vi "MeasureFastJoule.vi"(0 ".NET Refnum in":refnum<k24>, 1 ".NET Refnum":refnum<k24>, 2 "Junction Name":string, 5 "Maxiumum Voltage":dbl=8.0, 7 "appended path":path, 12 "new file path (Not A Path if cancelled)":path, 13 "UiDefinition":T1, 14 "Function":string) -> (15 "error out":errorcluster)   [LabVIEW 2020]
uses:
  D:/LabviewDXFViewer/LabviewDXFViewer/bin/Release/LabviewDXFViewer.exe
  LabviewDXFViewer/bin/Release/LabviewDXFViewer.exe
  UIReferences.ctl
  <vilib>/Utility/file.llb/Write Delimited Spreadsheet (string).vi
  <vilib>/Utility/file.llb/Write Delimited Spreadsheet (DBL).vi
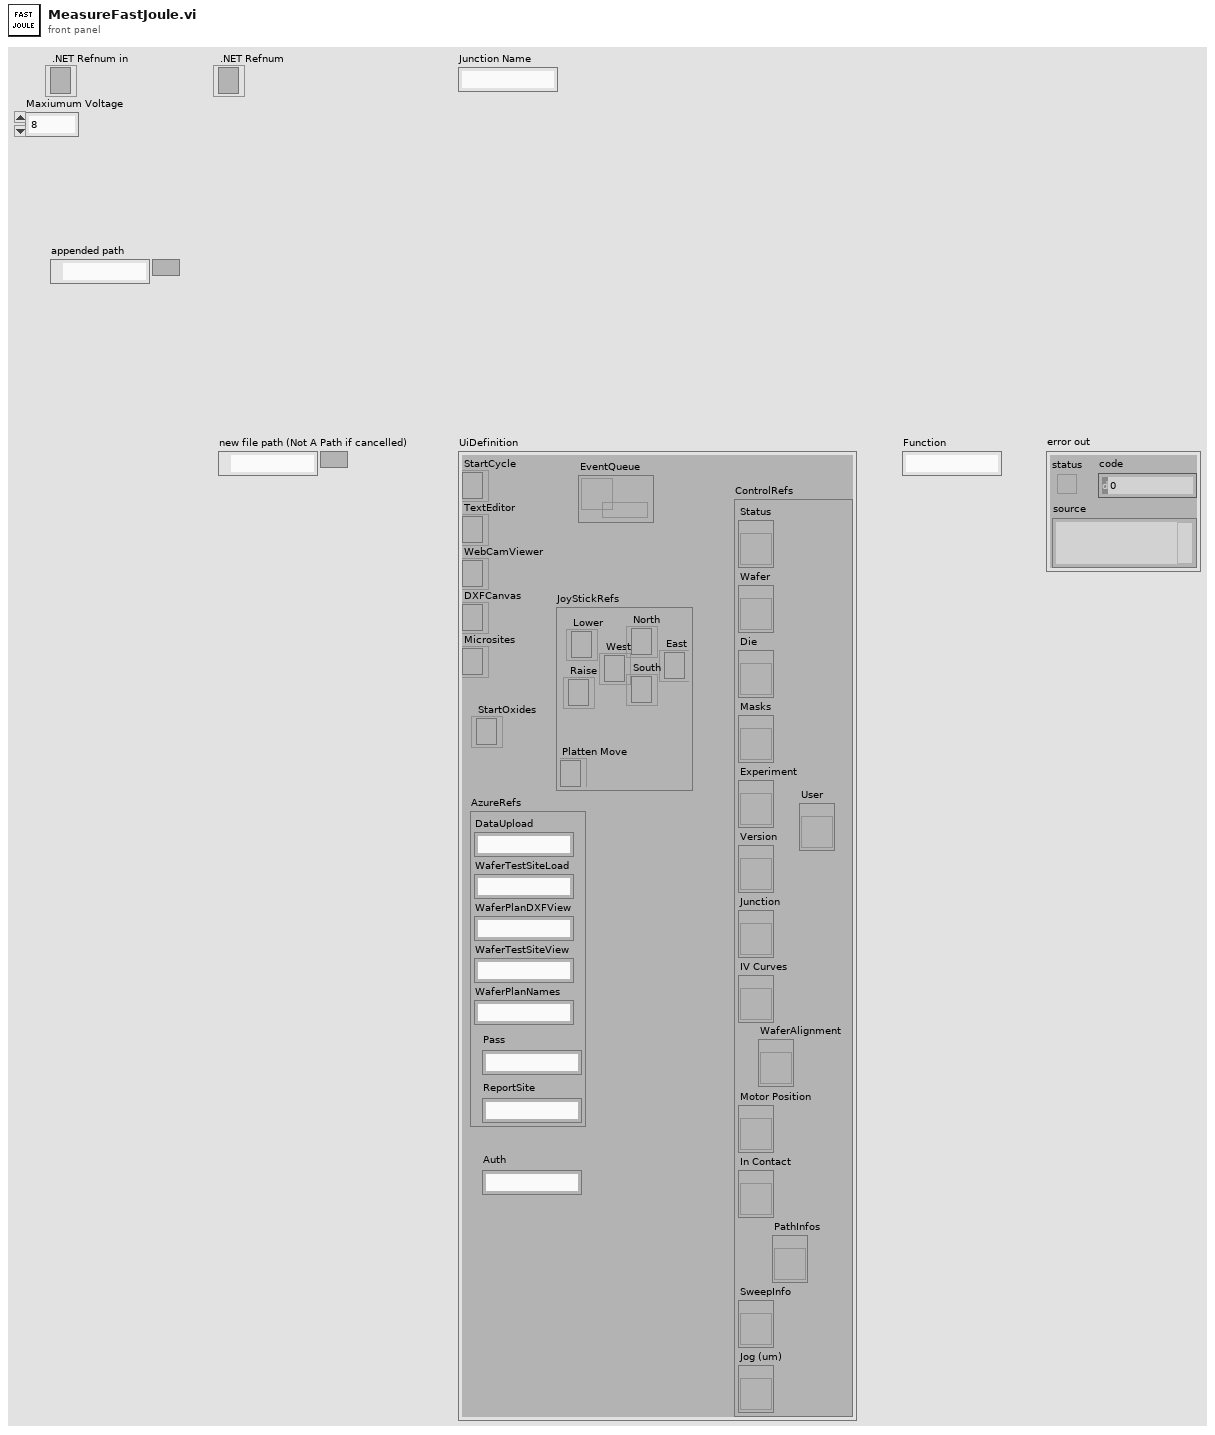
[diagram p1: front panel]
types:
  T1 = typedef "UIReferences.ctl" = cluster{"StartCycle":refnum<k24>, "TextEditor":refnum<k24>, "WebCamViewer":refnum<k24>, "DXFCanvas":refnum<k24>, "Microsites":refnum<k24>, "JoyStickRefs":cluster{"North":refnum<k24>, "Lower":refnum<k24>, "Raise":refnum<k24>, "Platten Move":refnum<k24>, "West":refnum<k24>, "East":refnum<k24>, "South":refnum<k24>}, "AzureRefs":cluster{"DataUpload":string, "WaferTestSiteLoad":string, "WaferPlanDXFView":string, "WaferTestSiteView":string, "WaferPlanNames":string, "Pass":string, "ReportSite":string}, "ControlRefs":cluster{"Status":refnum<vi>, "Wafer":refnum<vi>, "Die":refnum<vi>, "Masks":refnum<vi>, "Experiment":refnum<vi>, "Version":refnum<vi>, "Junction":refnum<vi>, "IV Curves":refnum<vi>, "Motor Position":refnum<vi>, "In Contact":refnum<vi>, "SweepInfo":refnum<vi>, "Jog (um)":refnum<vi>, "PathInfos":refnum<vi>, "User":refnum<vi>, "WaferAlignment":refnum<vi>}, "EventQueue":refnum<queue>, "StartOxides":refnum<k24>, "Auth":string}
  T2 = cluster{"Current Range":dbl, "Source Measure Unit Channel (0: Channel A)":i32, "Waveform":waveform(dbl), "VISA resource name":refnum<visa-resource-name>, "CodeText":string}
  T3 = typedef "CapacitanceInfos.ctl" = cluster{"Conductance":dbl, "CapacitanceIV":dbl, "Intercept":dbl, "CapacitanceSW":dbl, "Sum":dbl, "CapacitanceInfos":T4[], "CapacitancePhase":dbl, "dC/dV":dbl, "Function":string, "OtherInfo":dbl[][]}
  T4 = typedef "CapacitanceRecord.ctl" = cluster{"Freq":dbl, "Vpp":dbl, "PhaseS":dbl, "Irms":dbl, "PhaseC":dbl, "Theta":dbl, "VDrive":dbl, "Capacitance":dbl, "Other":dbl}
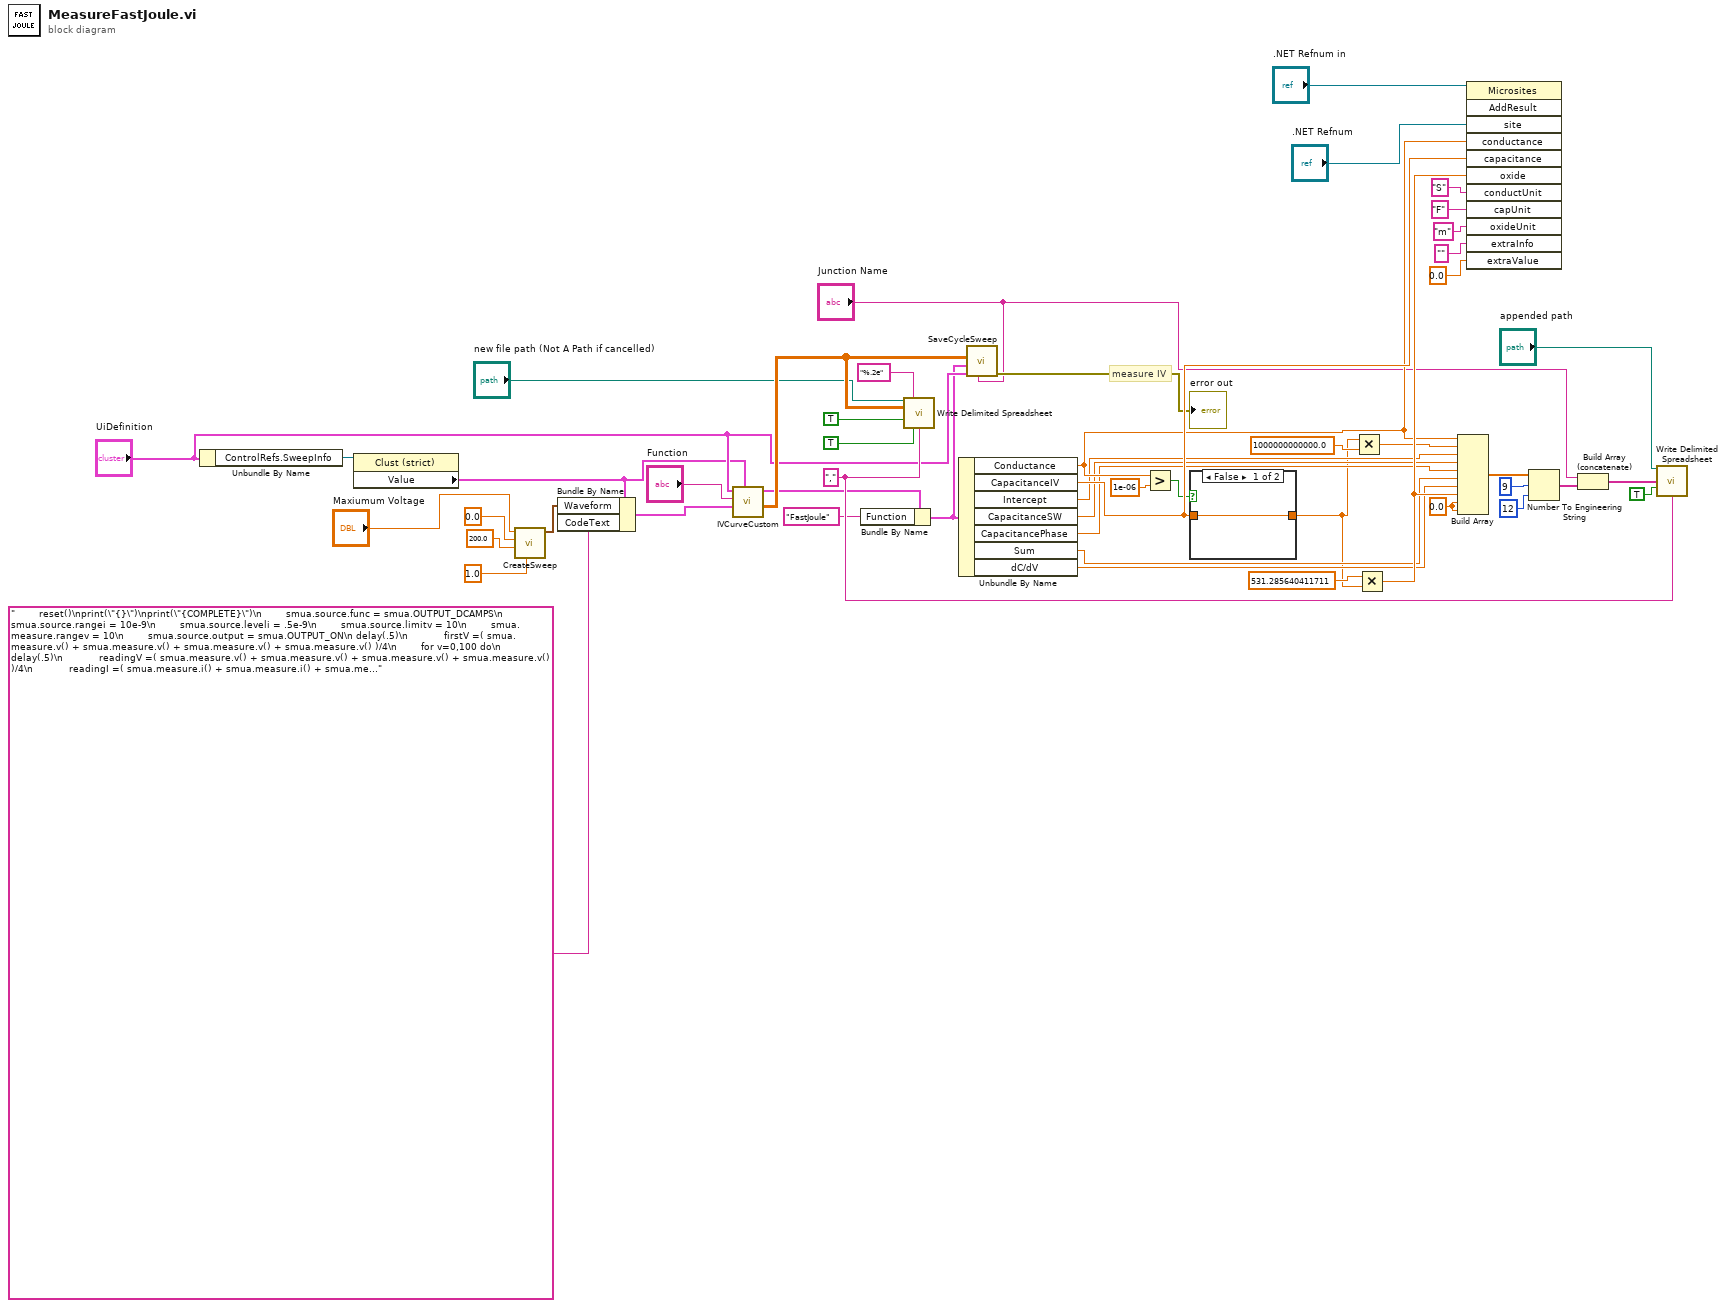
[diagram p0: block diagram]
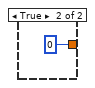
[diagram p2: hidden frame]
diagram:
  w4 = 0.0 ("element")
  w18 = "," ("delimiter (\\t)")
  # "measure IV"
  n1 = Unbundle By Name("UiDefinition") -> ("ControlRefs.SweepInfo"=w14:refnum<vi>)
  n2 = property class="Clust (strict)"(reference=w14) -> ("Value"=w1:T2)  [unwired: 1 in, 2 out]
  n3 = call "CreateSweep.vi"("Sweeps"=1.0, "Number Points"=200.0, "Minimum Voltage"=0.0, "Maxiumum Voltage"="Maxiumum Voltage") -> ("Waveform"=w12:waveform(dbl))  [unwired: 6 in, 1 out]
  n4 = Bundle By Name(cluster=w1, "Waveform"=w12, "CodeText"="        reset()\nprint(\"{}\")\nprint(\"{COMPLETE}\")\n        smua.source.func = smua.OUTPUT_DCAMPS\n        smua.source.rangei = 10e-9\n        smua.source.leveli = .5e-9\n        smua.source.limitv = 10\n        smua.measure.rangev = 10\n        smua.source.output = smua.OUTPUT_ON\n delay(.5)\n            firstV =( smua.measure.v() + smua.measure.v() + smua.measure.v() + smua.measure.v() )/4\n        for v=0,100 do\n            delay(.5)\n            readingV =( smua.measure.v() + smua.measure.v() + smua.measure.v() + smua.measure.v() )/4\n            readingI =( smua.measure.i() + smua.measure.i() + smua.measure.i() + smua.measure.i() )/4\n            time = os.date(\"*t\")\n            print(0, 1, 0,60*time.min+ time.sec , v*.5 , 0, 0,readingV,readingI)\nif (readingV>firstV*2) then break end\nif (readingV<firstV/2) then break end\nif (readingV>9) then break end\nif (readingV<.1) then break end\n        end\n\nsmua.source.rangei = 100e-9\n        smua.source.leveli = 10e-9\n        smua.source.limitv = 10\n        smua.measure.rangev = 10\n      \n delay(.5)\n            firstV =( smua.measure.v() + smua.measure.v() + smua.measure.v() + smua.measure.v() )/4\n        for v=0,50 do\n            delay(.5)\n            readingV =( smua.measure.v() + smua.measure.v() + smua.measure.v() + smua.measure.v() )/4\n            readingI =( smua.measure.i() + smua.measure.i() + smua.measure.i() + smua.measure.i() )/4\n            time = os.date(\"*t\")\n            print(0, 1, 0,60*time.min+ time.sec , v*.5 , 0, 0,readingV,readingI)\nif (readingV>firstV*2) then break end\nif (readingV<firstV/2) then break end\nif (readingV>9) then break end\nif (readingV<.1) then break end\n        end\n\n\nprint(\"{COMPLETE}\")\n\n        smua.source.output = smua.OUTPUT_OFF") -> (w13:T2)
  n5 = call "IVCurveCustom.vi"("OriginalSweepInfo"=w1, "SweepInfo"=w13, "Program"="Function", "UiDefinition"="UiDefinition") -> ("appended array"=w29:dbl[][], "InfoCluster"=w7:T3)  [unwired: 6 in]
  n6 = Bundle By Name(cluster=w7, "Function"="FastJoule") -> (w8:T3)
  n7 = call-poly <vilib>:"Write Delimited Spreadsheet.vi"("file path (dialog if empty)"="new file path (Not A Path if cancelled)", "format (%.3f)"="%.2e", "2D data"=w29, "append to file? (new file:F)"=TRUE, "transpose? (no:F)"=TRUE, "delimiter (\\t)"=w18) -> ()  [unwired: 8 in, 2 out]
  n8 = Unbundle By Name(w8) -> ("Conductance"=w48:dbl, "CapacitanceIV"=w49:dbl, "Intercept"=w32:dbl, "CapacitanceSW"=w37:dbl, "CapacitancePhase"=w38:dbl, "Sum"=w33:dbl, "dC/dV"=w34:dbl)
  n9 = call "SaveCycleSweep.vi"("JunctionName"="Junction Name", "UiDefinition 2"="UiDefinition", "InfoCluster"=w8, "appended array"=w29) -> ("error out"=→"error out":errorcluster)  [unwired: 7 in]
  n10 = Greater?(x=w48, y=1e-06) -> (0:w39:bool)
  n11 = case shown="False" w39 {
    tunnel: [w52 0] -> w16
    tunnel: w49 -> [w52 _]
    frame False {
    }
    frame True {
    }
  }
  n12 = Multiply(x=w16, y=1000000000000.0) -> (x*y=w35:dbl)
  n13 = Multiply(x=531.285640411711, y=w16) -> (x*y=w51:dbl)
  n14 = Build Array(w48, w35, w32, w37, w38, w33, w34, w51, w4, w4) -> (w31:dbl[])
  n15 = invoke class="Microsites" method="AddResult"(reference=".NET Refnum in", "site"=".NET Refnum", "conductance"=w48, "capacitance"=w49, "oxide"=w51, "conductUnit"="S", "capUnit"="F", "oxideUnit"="m" ("interceptUnit"), "extraInfo"="", "extraValue"=0.0) -> ()  [unwired: 2 in, 12 out]
  n16 = Number To Engineering String(2:i16 12 ("precision (6)"), 3:i16 9 ("width (-)"), 4:w31) -> (0:w23:string[])  [unwired: 1 in]
  n17 = Build Array (concatenate)("Junction Name", w23) -> (w25:string[])
  n18 = call-poly <vilib>:"Write Delimited Spreadsheet.vi"("file path (dialog if empty)"="appended path", "1D data"=w25, "append to file? (new file:F)"=TRUE, "delimiter (\\t)"=w18) -> ()  [unwired: 10 in, 2 out]
